vi "Stop.vi"   [LabVIEW 2019]
uses:
  <vilib>/rvi/eio/common/nirviEmuTemplateMethod_errors.vi
  <vilib>/eio/EIONode/EIONode.xnode
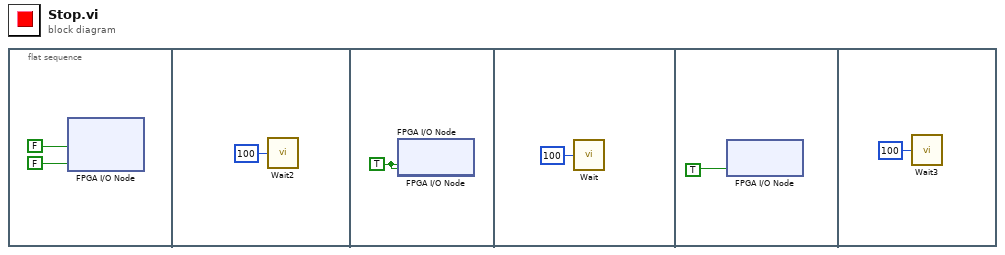
[diagram p0: block diagram]
diagram:
  n1 = flat-sequence {
    frame #0 {
      n2 = xnode "FPGA I/O Node"("SDA"=FALSE, "SCL"=FALSE) -> ()  [unwired: 2 in, 2 out]
    }
    frame #1 {
      n3 = call "Wait2"("Count(mSec)"=u32 100) -> ()  [unwired: 1 out]
    }
    frame #2 {
      w4 = TRUE ("SDA")
      n4 = xnode "FPGA I/O Node"("SDA"=w4) -> ()  [unwired: 1 in, 1 out]
      n5 = xnode "FPGA I/O Node"("SCL"=w4) -> ()  [unwired: 1 in, 1 out]
    }
    frame #3 {
      n6 = call "Wait"("Count(mSec)"=u32 100) -> ()  [unwired: 1 out]
    }
    frame #4 {
      n7 = xnode "FPGA I/O Node"("SDA"=TRUE) -> ()  [unwired: 1 in, 1 out]
    }
    frame #5 {
      n8 = call "Wait3"("Count(mSec)"=u32 100) -> ()  [unwired: 1 out]
    }
  }
